vi "todatacluster.vi"(10 "ROI":T4, 11 "Images":T3) -> (3 "data":T1)   [LabVIEW 2011]
uses:
  ROIStartfromCam_typdef.ctl
  analysis_data_typdef.ctl
  IMAQ Image.ctl
  dataTypdef.ctl
  MagAnalysis_Online.lvclass
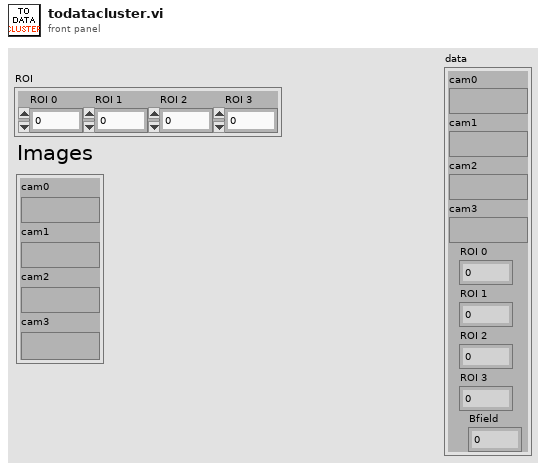
[diagram p1: front panel]
types:
  T1 = typedef "dataTypdef.ctl" = cluster{"cam0":T2, "cam1":T2, "cam2":T2, "cam3":T2, "ROI 0":dbl, "ROI 1":dbl, "ROI 2":dbl, "ROI 3":dbl, "Bfield":dbl}
  T2 = typedef "IMAQ Image.ctl" = refnum<image>
  T3 = typedef "MagAnalysis_Online.lvclass/analysis_data_typdef.ctl" = cluster{"cam0":T2, "cam1":T2, "cam2":T2, "cam3":T2}
  T4 = typedef "ROIStartfromCam_typdef.ctl" = cluster{"ROI 0":dbl, "ROI 1":dbl, "ROI 2":dbl, "ROI 3":dbl}
  T5 = cluster{"cam0":T2, "cam1":T2, "cam2":T2, "cam3":T2, "ROI 0":dbl, "ROI 1":dbl, "ROI 2":dbl, "ROI 3":dbl, "B[mT]":dbl}
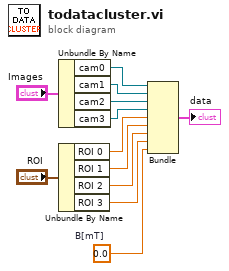
[diagram p0: block diagram]
diagram:
  w1 = 0.0  # B[mT]
  n1 = Unbundle By Name("Images") -> ("cam0"=w10:T2, "cam1"=w9:T2, "cam2"=w8:T2, "cam3"=w7:T2)
  n2 = Unbundle By Name("ROI") -> ("ROI 0"=w6:dbl, "ROI 1"=w5:dbl, "ROI 2"=w4:dbl, "ROI 3"=w3:dbl)
  n3 = Bundle("cam0"=w10, "cam1"=w9, "cam2"=w8, "cam3"=w7, "ROI 0"=w6, "ROI 1"=w5, "ROI 2"=w4, "ROI 3"=w3, "B[mT]"=w1) -> (→"data":T5)  [unwired: 1 in]
